vi "Driver Station Status Message.vi"(10 "Message":string, 11 "Message Type":enum16{"Error", "Warning", "Info"}(ring)) -> ()   [LabVIEW 2016]
uses:
  Robot Global Data.vi
  <vilib>/Rock Robotics/Network Tables/NT Write String.vi
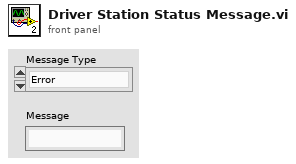
[diagram p1: front panel]
types:
  T1 = typedef "WPI_DriverStationRobotMode2.ctl" = enum16{"Autonomous Disabled", "Autonomous Enabled", "Teleop Disabled", "Teleop Enabled", "Disconnected", "Finish", "Test Disabled", "Test Enabled", "Emergency Stopped"}
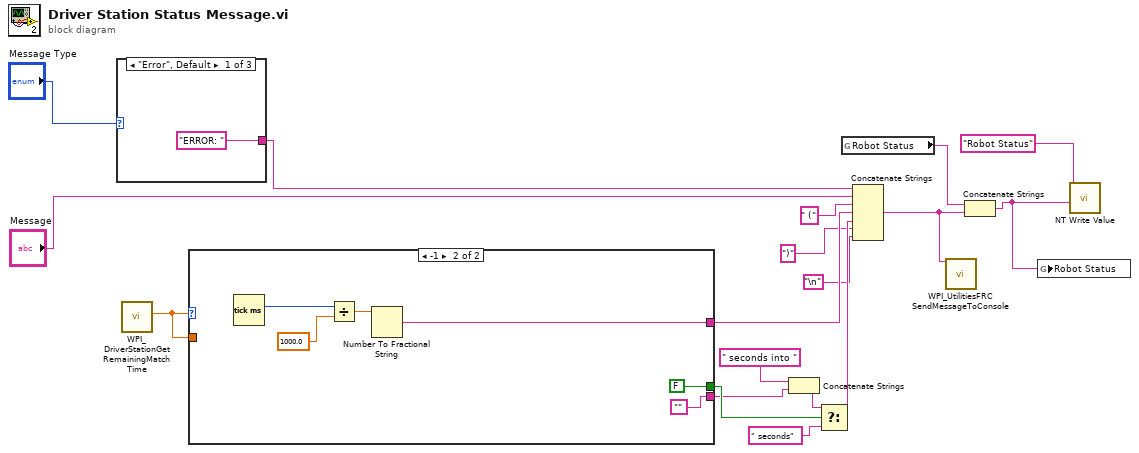
[diagram p0: block diagram]
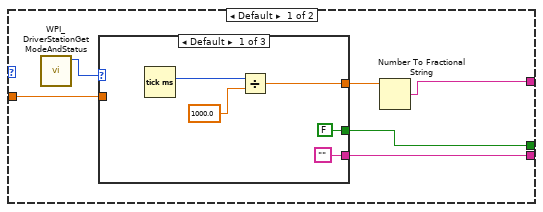
[diagram p2: hidden frame]
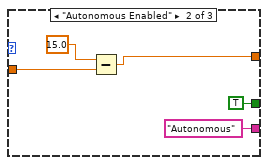
[diagram p3: hidden frame]
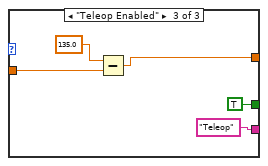
[diagram p4: hidden frame]
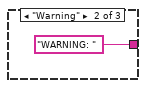
[diagram p5: hidden frame]
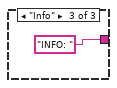
[diagram p6: hidden frame]
diagram:
  n1 = case shown="\"Error\", Default" "Message Type" {
    tunnel: ["ERROR: " ("string") "WARNING: " ("string") "INFO: " ("string")] -> w15
    frame "Error", Default {
    }
    frame "Warning" {
    }
    frame "Info" {
    }
  }
  n2 = call <vilib>:"WPI_DriverStationGetRemainingMatchTime.vi"() -> ("Match Time(s)"=w17:sgl)  [unwired: 10 in, 1 out]
  n3 = case shown="-1" w17 {
    tunnel: w17 -> [w26 _]
    tunnel: [w24 FALSE] -> w16
    tunnel: [w23 w44] -> w12
    tunnel: [w22 ""] -> w6
    frame Default {
      n4 = call <vilib>:"WPI_DriverStationGetModeAndStatus.vi"() -> ("Robot Mode"=w27:T1)  [unwired: 10 in, 1 out]
      n5 = case shown="Default" w27 {
        tunnel: w26 -> [_ w36 w41]
        tunnel: [w30 w35 w40] -> w25
        tunnel: [FALSE TRUE TRUE] -> w24
        tunnel: ["" "Autonomous" "Teleop"] -> w22
        frame Default {
          n6 = Tick Count (ms)() -> (millisecond timer value=w32:u32)
          n7 = Divide(x=w32, y=1000.0) -> (x/y=w30:dbl)
        }
        frame "Autonomous Enabled" {
          n8 = Subtract(x=15.0, y=w36) -> (x-y=w35:dbl)
        }
        frame "Teleop Enabled" {
          n9 = Subtract(x=135.0, y=w41) -> (x-y=w40:dbl)
        }
      }
      n10 = Number To Fractional String(number=w25) -> (F-format string=w23:string)  [unwired: 3 in]
    }
    frame -1 {
      n11 = Tick Count (ms)() -> (millisecond timer value=w48:u32)
      n12 = Divide(x=w48, y=1000.0) -> (x/y=w46:dbl)
      n13 = Number To Fractional String(number=w46) -> (F-format string=w44:string)  [unwired: 3 in]
    }
  }
  n14 = Concatenate Strings(" seconds into ", w6) -> (w8:string)
  n15 = Select(t=w8, s=w16, f=" seconds") -> (s? t:f=w11:string)
  n16 = global read "Robot Global Data.vi" "Robot Status"() -> (w4:string)
  n17 = Concatenate Strings(w15, "Message", " (" ("string"), w12, w11, ")" ("string"), "\n") -> (w1:string)
  n18 = call <vilib>:"WPI_UtilitiesFRC SendMessageToConsole.vi"("Message"=w1) -> ()  [unwired: 14 in, 1 out]
  n19 = Concatenate Strings(w4, w1) -> (w2:string)
  n20 = global write "Robot Global Data.vi" "Robot Status"(w2) -> ()
  n21 = call-poly <vilib>:"NT Write Value.vi"("String"=w2, "Name"="Robot Status") -> ()  [unwired: 9 in, 1 out]
